vi "Cycle Diag Table Read.vi"(5 "Raw Data In":string) -> (4 "output cluster":T1)   [LabVIEW 2016, in "2015 VA Washer.lvlib"]
uses:
  Projects/2015 VA Washer.lvlib
  type defs/Cycle_Diag_Teststand.ctl
panel:
  out "appended array":string[](array[string])
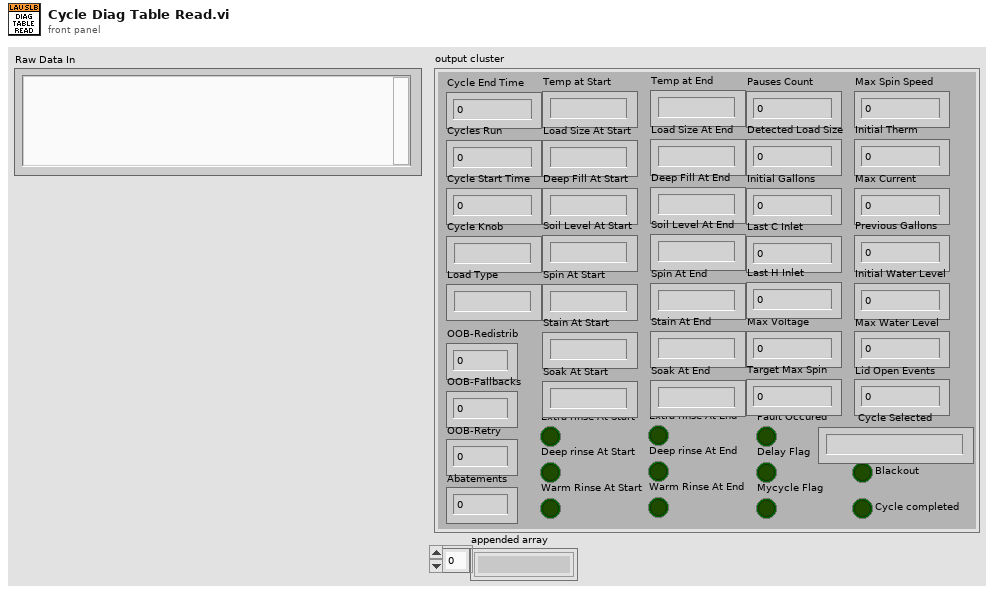
[diagram p1: front panel]
types:
  T1 = typedef "2015 VA Washer.lvlib/Cycle_Diag_Teststand.ctl" = cluster{"Cycle End Time":u32, "Cycles Run":u32, "Cycle Start Time":u32, "Cycle Knob":string, "Load Type":string, "OOB-Redistrib":u8, "OOB-Fallbacks":u8, "OOB-Retry":u8, "Temp at Start":string, "Load Size At Start":string, "Deep Fill At Start":string, "Soil Level At Start":string, "Spin At Start":string, "Extra rinse At Start":bool, "Deep rinse At Start":bool, "Stain At Start":string, "Soak At Start":string, "Warm Rinse At Start":bool, "Temp at End":string, "Load Size At End":string, "Deep Fill At End":string, "Soil Level At End":string, "Spin At End":string, "Extra rinse At End":bool, "Deep rinse At End":bool, "Stain At End":string, "Soak At End":string, "Warm Rinse At End":bool, "Pauses Count":u8, "Fault Occured":bool, "Delay Flag":bool, "Mycycle Flag":bool, "Blackout":bool, "Cycle completed":bool, "Detected Load Size":dbl, "Initial Gallons":dbl, "Last C Inlet ":dbl, "Max Voltage":dbl, "Target Max Spin":u16, "Max Spin Speed":u16, "Initial Therm":dbl, "Max Current":dbl, "Previous Gallons":dbl, "Initial Water Level":dbl, "Max Water Level":dbl, "Abatements ":u8, "Lid Open Events":u8, "Cycle Selected":string, "Last H Inlet ":dbl}
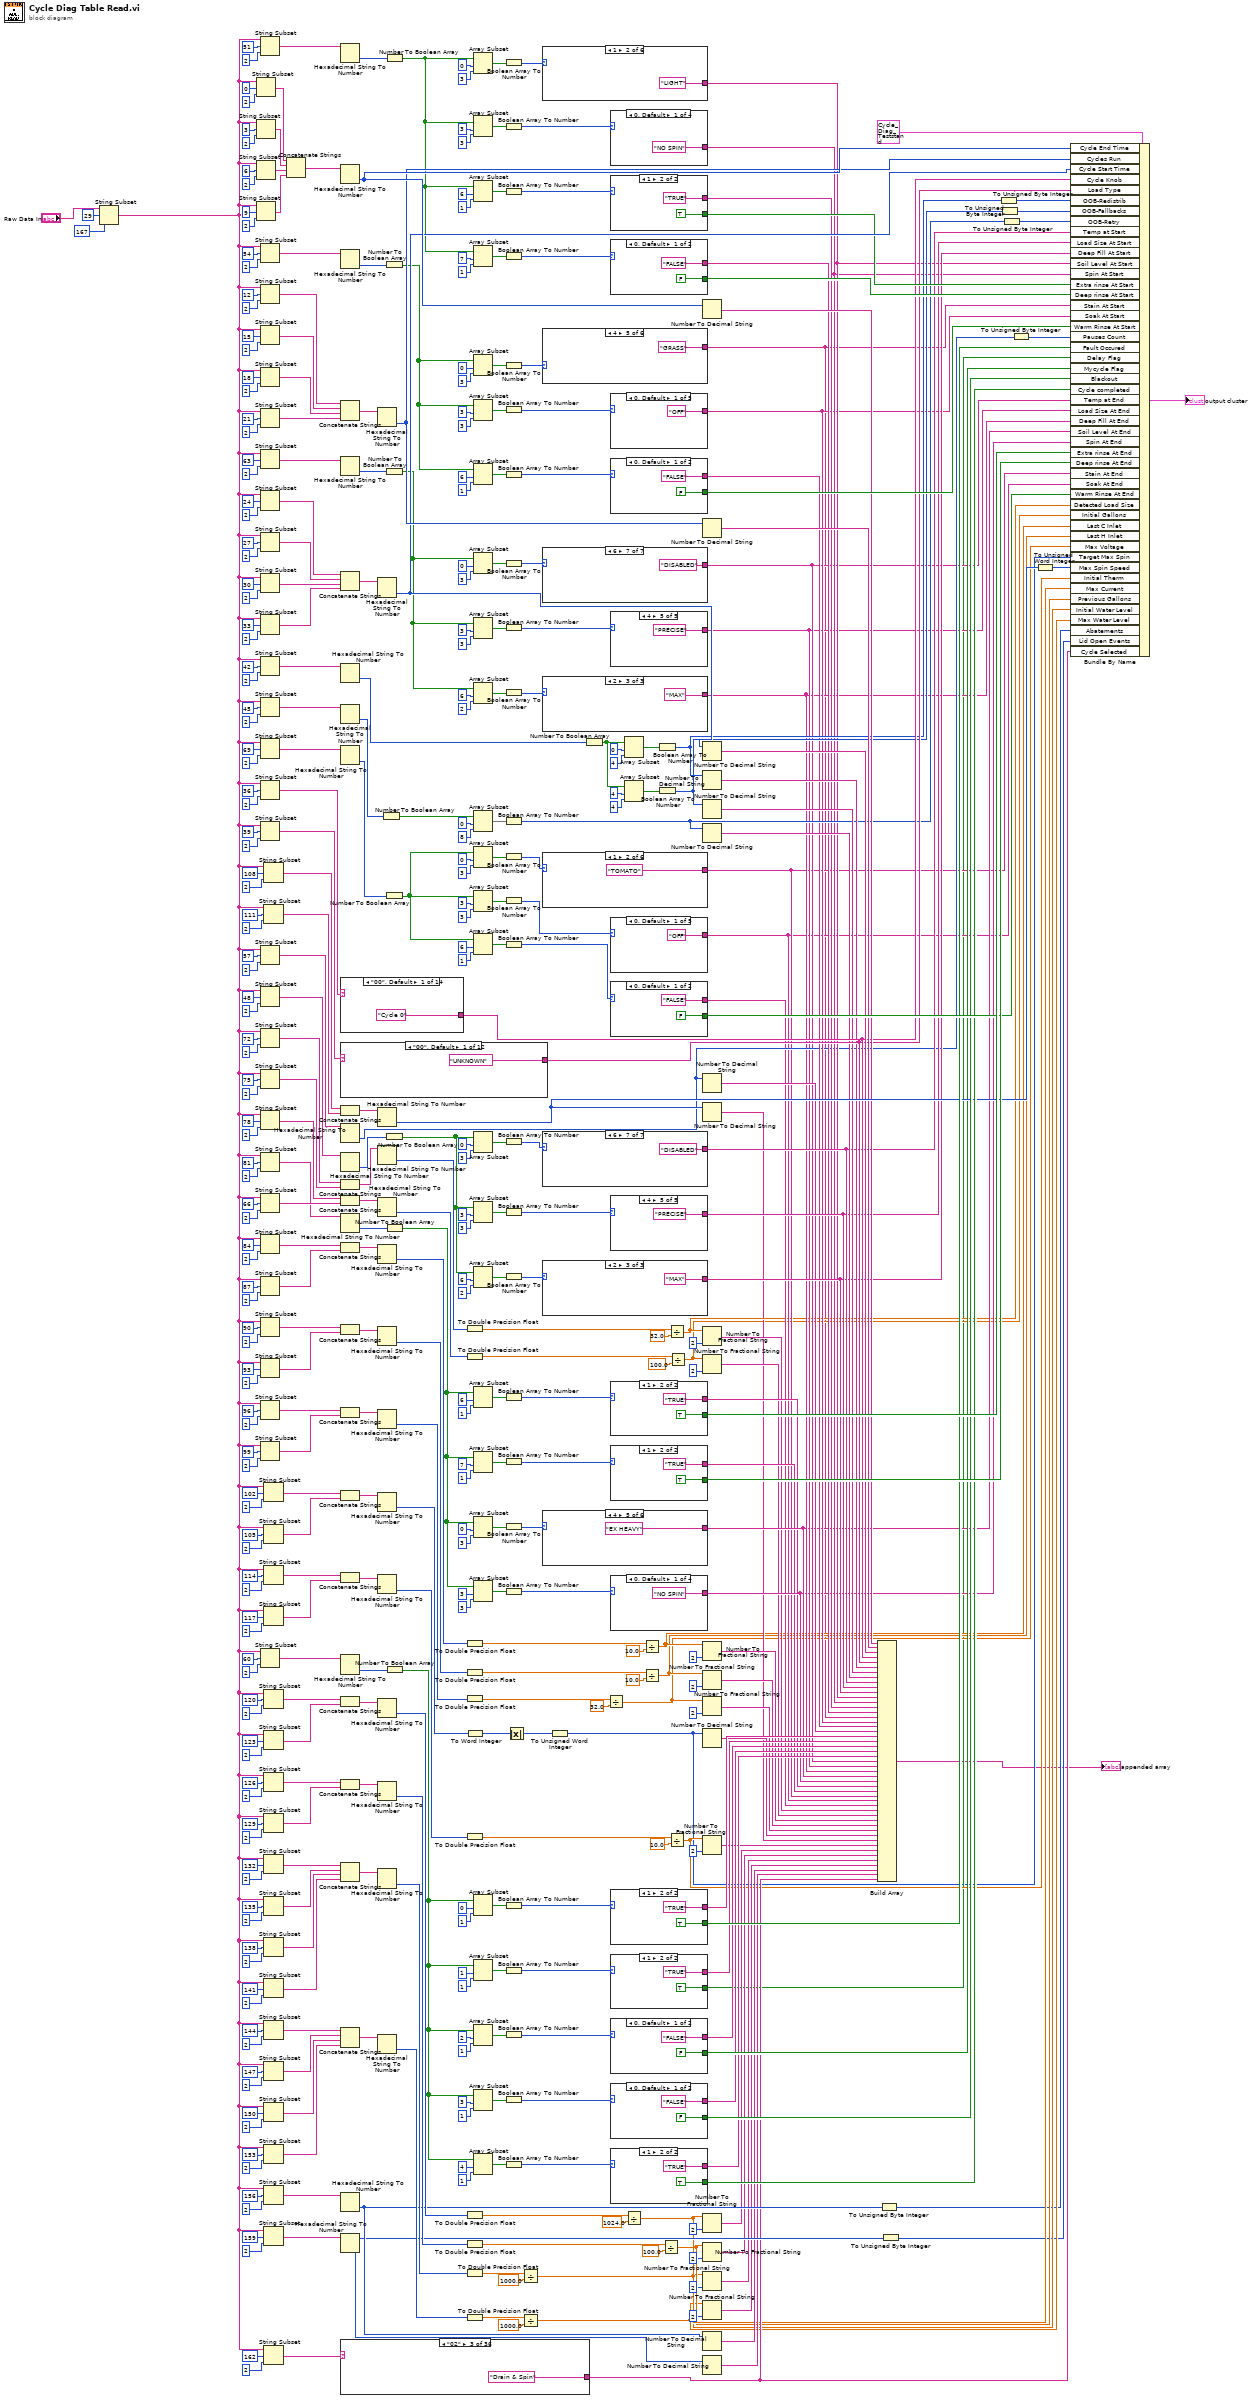
[diagram p0: block diagram]
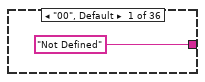
[diagram p2: hidden frame]
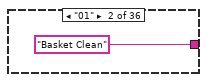
[diagram p3: hidden frame]
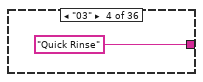
[diagram p4: hidden frame]
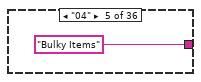
[diagram p5: hidden frame]
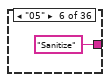
[diagram p6: hidden frame]
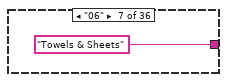
[diagram p7: hidden frame]
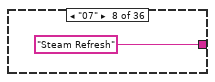
[diagram p8: hidden frame]
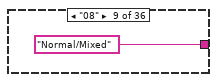
[diagram p9: hidden frame]
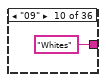
[diagram p10: hidden frame]
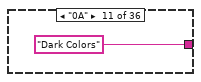
[diagram p11: hidden frame]
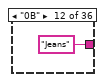
[diagram p12: hidden frame]
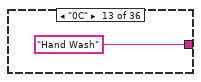
[diagram p13: hidden frame]
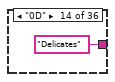
[diagram p14: hidden frame]
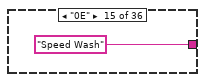
[diagram p15: hidden frame]
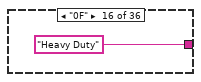
[diagram p16: hidden frame]
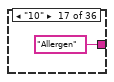
[diagram p17: hidden frame]
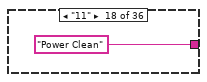
[diagram p18: hidden frame]
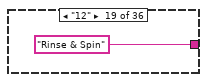
[diagram p19: hidden frame]
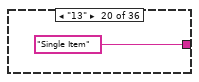
[diagram p20: hidden frame]
diagram:
  n1 = String Subset(string="Raw Data In", offset (0)=29, length (rest)=167 ("length (rest)")) -> (substring=w4:string)
  n2 = String Subset(string=w4, offset (0)=0, length (rest)=2 ("length (rest)")) -> (substring=w413:string)
  n3 = String Subset(string=w4, offset (0)=3, length (rest)=2 ("length (rest)")) -> (substring=w412:string)
  n4 = String Subset(string=w4, offset (0)=6, length (rest)=2 ("length (rest)")) -> (substring=w411:string)
  n5 = String Subset(string=w4, offset (0)=9, length (rest)=2 ("length (rest)")) -> (substring=w410:string)
  n6 = String Subset(string=w4, offset (0)=51, length (rest)=2 ("length (rest)")) -> (substring=w116:string)
  n7 = String Subset(string=w4, offset (0)=54, length (rest)=2 ("length (rest)")) -> (substring=w100:string)
  n8 = String Subset(string=w4, offset (0)=12, length (rest)=2 ("length (rest)")) -> (substring=w407:string)
  n9 = String Subset(string=w4, offset (0)=15, length (rest)=2 ("length (rest)")) -> (substring=w406:string)
  n10 = String Subset(string=w4, offset (0)=18, length (rest)=2 ("length (rest)")) -> (substring=w405:string)
  n11 = String Subset(string=w4, offset (0)=21, length (rest)=2 ("length (rest)")) -> (substring=w404:string)
  n12 = String Subset(string=w4, offset (0)=63, length (rest)=2 ("length (rest)")) -> (substring=w87:string)
  n13 = String Subset(string=w4, offset (0)=24, length (rest)=2 ("length (rest)")) -> (substring=w401:string)
  n14 = String Subset(string=w4, offset (0)=27, length (rest)=2 ("length (rest)")) -> (substring=w400:string)
  n15 = String Subset(string=w4, offset (0)=30, length (rest)=2 ("length (rest)")) -> (substring=w399:string)
  n16 = String Subset(string=w4, offset (0)=33, length (rest)=2 ("length (rest)")) -> (substring=w398:string)
  n17 = String Subset(string=w4, offset (0)=42, length (rest)=2 ("length (rest)")) -> (substring=w56:string)
  n18 = String Subset(string=w4, offset (0)=45, length (rest)=2 ("length (rest)")) -> (substring=w47:string)
  n19 = String Subset(string=w4, offset (0)=69, length (rest)=2 ("length (rest)")) -> (substring=w60:string)
  n20 = String Subset(string=w4, offset (0)=36, length (rest)=2 ("length (rest)")) -> (substring=w395:string)
  n21 = String Subset(string=w4, offset (0)=39, length (rest)=2 ("length (rest)")) -> (substring=w394:string)
  n22 = String Subset(string=w4, offset (0)=57, length (rest)=2 ("length (rest)")) -> (substring=w352:string)
  n23 = String Subset(string=w4, offset (0)=48, length (rest)=2 ("length (rest)")) -> (substring=w135:string)
  n24 = String Subset(string=w4, offset (0)=72, length (rest)=2 ("length (rest)")) -> (substring=w336:string)
  n25 = String Subset(string=w4, offset (0)=75 ("offset"), length (rest)=u32 2 ("default (0 U32)")) -> (substring=w333:string)
  n26 = String Subset(string=w4, offset (0)=78, length (rest)=2 ("length (rest)")) -> (substring=w328:string)
  n27 = String Subset(string=w4, offset (0)=81, length (rest)=2 ("length (rest)")) -> (substring=w327:string)
  n28 = String Subset(string=w4, offset (0)=66, length (rest)=2 ("length (rest)")) -> (substring=w73:string)
  n29 = String Subset(string=w4, offset (0)=84, length (rest)=2 ("length (rest)")) -> (substring=w317:string)
  n30 = String Subset(string=w4, offset (0)=87, length (rest)=2 ("length (rest)")) -> (substring=w316:string)
  n31 = String Subset(string=w4, offset (0)=90, length (rest)=2 ("length (rest)")) -> (substring=w311:string)
  n32 = String Subset(string=w4, offset (0)=93, length (rest)=2 ("length (rest)")) -> (substring=w310:string)
  n33 = String Subset(string=w4, offset (0)=96, length (rest)=2 ("length (rest)")) -> (substring=w301:string)
  n34 = String Subset(string=w4, offset (0)=99, length (rest)=2 ("length (rest)")) -> (substring=w300:string)
  n35 = String Subset(string=w4, offset (0)=60, length (rest)=2 ("length (rest)")) -> (substring=w351:string)
  n36 = String Subset(string=w4, offset (0)=108, length (rest)=2 ("length (rest)")) -> (substring=w288:string)
  n37 = String Subset(string=w4, offset (0)=111, length (rest)=2 ("length (rest)")) -> (substring=w287:string)
  n38 = String Subset(string=w4, offset (0)=102, length (rest)=2 ("length (rest)")) -> (substring=w291:string)
  n39 = String Subset(string=w4, offset (0)=105, length (rest)=2 ("length (rest)")) -> (substring=w290:string)
  n40 = String Subset(string=w4, offset (0)=114, length (rest)=2 ("length (rest)")) -> (substring=w276:string)
  n41 = String Subset(string=w4, offset (0)=117, length (rest)=2 ("length (rest)")) -> (substring=w275:string)
  n42 = String Subset(string=w4, offset (0)=120, length (rest)=2 ("length (rest)")) -> (substring=w266:string)
  n43 = String Subset(string=w4, offset (0)=123, length (rest)=2 ("length (rest)")) -> (substring=w265:string)
  n44 = String Subset(string=w4, offset (0)=126, length (rest)=2 ("length (rest)")) -> (substring=w256:string)
  n45 = String Subset(string=w4, offset (0)=129, length (rest)=2 ("length (rest)")) -> (substring=w255:string)
  n46 = String Subset(string=w4, offset (0)=132, length (rest)=2 ("length (rest)")) -> (substring=w246:string)
  n47 = String Subset(string=w4, offset (0)=135, length (rest)=2 ("length (rest)")) -> (substring=w245:string)
  n48 = String Subset(string=w4, offset (0)=138, length (rest)=2 ("length (rest)")) -> (substring=w215:string)
  n49 = String Subset(string=w4, offset (0)=141, length (rest)=2 ("length (rest)")) -> (substring=w214:string)
  n50 = String Subset(string=w4, offset (0)=144, length (rest)=2 ("length (rest)")) -> (substring=w240:string)
  n51 = String Subset(string=w4, offset (0)=147, length (rest)=2 ("length (rest)")) -> (substring=w239:string)
  n52 = String Subset(string=w4, offset (0)=150, length (rest)=2 ("length (rest)")) -> (substring=w209:string)
  n53 = String Subset(string=w4, offset (0)=153, length (rest)=2 ("length (rest)")) -> (substring=w208:string)
  n54 = String Subset(string=w4, offset (0)=156, length (rest)=2 ("length (rest)")) -> (substring=w220:string)
  n55 = String Subset(string=w4, offset (0)=159, length (rest)=2 ("length (rest)")) -> (substring=w219:string)
  n56 = String Subset(string=w4, offset (0)=162, length (rest)=2 ("length (rest)")) -> (substring=w216:string)
  n57 = Concatenate Strings(w413, w412, w411, w410) -> (w409:string)
  n58 = Hexadecimal String To Number(string=w116) -> (number=w123:u32)  [unwired: 2 in, 1 out]
  n59 = Hexadecimal String To Number(string=w409) -> (number=w408:u32)  [unwired: 2 in, 1 out]
  n60 = Hexadecimal String To Number(string=w100) -> (number=w108:u32)  [unwired: 2 in, 1 out]
  n61 = Concatenate Strings(w407, w406, w405, w404) -> (w403:string)
  n62 = Hexadecimal String To Number(string=w87) -> (number=w95:u32)  [unwired: 2 in, 1 out]
  n63 = Concatenate Strings(w401, w400, w399, w398) -> (w397:string)
  n64 = Hexadecimal String To Number(string=w56) -> (number=w55:u32)  [unwired: 2 in, 1 out]
  n65 = Hexadecimal String To Number(string=w47) -> (number=w46:u32)  [unwired: 2 in, 1 out]
  n66 = Hexadecimal String To Number(string=w60) -> (number=w68:u32)  [unwired: 2 in, 1 out]
  n67 = case shown="\"00\", Default" w395 {
    tunnel: ["Cycle 0" "Cycle 1" "Cycle 2" "Cycle 3" "Cycle 4" "Cycle 5" "Cycle 6" "Cycle 7" "Cycle 8" "Cycle 9" "Cycle 10" "Cycle 11" "Cycle 12" "Cycle 13"] -> w196
    frame "00", Default {
    }
    frame "01" {
    }
    frame "02" {
    }
    frame "03" {
    }
    frame "04" {
    }
    frame "05" {
    }
    frame "06" {
    }
    frame "07" {
    }
    frame "08" {
    }
    frame "09" {
    }
    frame "0A" {
    }
    frame "0B" {
    }
    frame "0C" {
    }
    frame "0D" {
    }
  }
  n68 = case shown="\"00\", Default" w394 {
    tunnel: ["UNKNOWN" "COTTON" "SYNTHETIC" "MIXED" "WET" "LOW FLOW" "SMALL" "MEDIUM" "LARGE" "SUPER" "SUPER PLUS" "MAX"] -> w195
    frame "00", Default {
    }
    frame "01" {
    }
    frame "02" {
    }
    frame "03" {
    }
    frame "04" {
    }
    frame "05" {
    }
    frame "06" {
    }
    frame "07" {
    }
    frame "08" {
    }
    frame "09" {
    }
    frame "0A" {
    }
    frame "0B" {
    }
  }
  n69 = Concatenate Strings(w288, w287) -> (w286:string)
  n70 = Hexadecimal String To Number(string=w352) -> (number=w179:u32)  [unwired: 2 in, 1 out]
  n71 = Hexadecimal String To Number(string=w135) -> (number=w134:u32)  [unwired: 2 in, 1 out]
  n72 = Concatenate Strings(w336, w333) -> (w332:string)
  n73 = Concatenate Strings(w328, w327) -> (w326:string)
  n74 = Hexadecimal String To Number(string=w73) -> (number=w83:u32)  [unwired: 2 in, 1 out]
  n75 = Concatenate Strings(w317, w316) -> (w315:string)
  n76 = Concatenate Strings(w311, w310) -> (w309:string)
  n77 = Concatenate Strings(w301, w300) -> (w299:string)
  n78 = Concatenate Strings(w291, w290) -> (w289:string)
  n79 = Concatenate Strings(w276, w275) -> (w274:string)
  n80 = Hexadecimal String To Number(string=w351) -> (number=w350:u32)  [unwired: 2 in, 1 out]
  n81 = Concatenate Strings(w266, w265) -> (w264:string)
  n82 = Concatenate Strings(w256, w255) -> (w254:string)
  n83 = Concatenate Strings(w246, w245, w215, w214) -> (w244:string)
  n84 = Concatenate Strings(w240, w239, w209, w208) -> (w238:string)
  n85 = Hexadecimal String To Number(string=w220) -> (number=w218:u32)  [unwired: 2 in, 1 out]
  n86 = Hexadecimal String To Number(string=w219) -> (number=w217:u32)  [unwired: 2 in, 1 out]
  n87 = case shown="\"02\"" w216 {
    tunnel: ["Not Defined" "Basket Clean" "Drain & Spin" "Quick Rinse" "Bulky Items" "Sanitize" "Towels & Sheets" "Steam Refresh" "Normal/Mixed" "Whites" "Dark Colors" "Jeans" "Hand Wash" "Delicates" "Speed Wash" "Heavy Duty" "Allergen" "Power Clean" "Rinse & Spin" "Single Item" "Colors" "Cold Wash" "Cottons" "Easy Care" "Active Wear" "Timed Dry" "Dewrinkle" "Air Fluff" "Steam Refresh" "Steam Dewrinkle" "Speed Dry" "Mixed" "Quick Dry" "Casuals" "Warm Up" "Energy Saver"] -> w146
    frame "00", Default {
    }
    frame "01" {
    }
    frame "02" {
    }
    frame "03" {
    }
    frame "04" {
    }
    frame "05" {
    }
    frame "06" {
    }
    frame "07" {
    }
    frame "08" {
    }
    frame "09" {
    }
    frame "0A" {
    }
    frame "0B" {
    }
    frame "0C" {
    }
    frame "0D" {
    }
    frame "0E" {
    }
    frame "0F" {
    }
    frame "10" {
    }
    frame "11" {
    }
    frame "12" {
    }
    frame "13" {
    }
    frame "14" {
    }
    frame "15" {
    }
    frame "80" {
    }
    frame "81" {
    }
    frame "82" {
    }
    frame "83" {
    }
    frame "84" {
    }
    frame "85" {
    }
    frame "86" {
    }
    frame "87" {
    }
    frame "88" {
    }
    frame "89" {
    }
    frame "8A" {
    }
    frame "8B" {
    }
    frame "8C" {
    }
    frame "8D" {
    }
  }
  n88 = Hexadecimal String To Number(string=w403) -> (number=w402:u32)  [unwired: 2 in, 1 out]
  n89 = Hexadecimal String To Number(string=w397) -> (number=w396:u32)  [unwired: 2 in, 1 out]
  n90 = Hexadecimal String To Number(string=w286) -> (number=w285:u32)  [unwired: 2 in, 1 out]
  n91 = Hexadecimal String To Number(string=w332) -> (number=w339:u32)  [unwired: 2 in, 1 out]
  n92 = Hexadecimal String To Number(string=w326) -> (number=w325:u32)  [unwired: 2 in, 1 out]
  n93 = Hexadecimal String To Number(string=w315) -> (number=w314:u32)  [unwired: 2 in, 1 out]
  n94 = Hexadecimal String To Number(string=w309) -> (number=w308:u32)  [unwired: 2 in, 1 out]
  n95 = Hexadecimal String To Number(string=w299) -> (number=w298:u32)  [unwired: 2 in, 1 out]
  n96 = Hexadecimal String To Number(string=w289) -> (number=w201:u32)  [unwired: 2 in, 1 out]
  n97 = Hexadecimal String To Number(string=w274) -> (number=w273:u32)  [unwired: 2 in, 1 out]
  n98 = Hexadecimal String To Number(string=w264) -> (number=w263:u32)  [unwired: 2 in, 1 out]
  n99 = Hexadecimal String To Number(string=w254) -> (number=w253:u32)  [unwired: 2 in, 1 out]
  n100 = Hexadecimal String To Number(string=w244) -> (number=w243:u32)  [unwired: 2 in, 1 out]
  n101 = Hexadecimal String To Number(string=w238) -> (number=w237:u32)  [unwired: 2 in, 1 out]
  n102 = Number To Boolean Array(number=w46) -> (Boolean array=w45:bool[])
  n103 = Number To Boolean Array(number=w108) -> (Boolean array=w107:bool[])
  n104 = Number To Boolean Array(number=w95) -> (Boolean array=w94:bool[])
  n105 = Number To Boolean Array(number=w68) -> (Boolean array=w67:bool[])
  n106 = Number To Boolean Array(number=w134) -> (Boolean array=w133:bool[])
  n107 = Number To Boolean Array(number=w123) -> (Boolean array=w115:bool[])
  n108 = Number To Boolean Array(number=w83) -> (Boolean array=w76:bool[])
  n109 = Number To Boolean Array(number=w350) -> (Boolean array=w31:bool[])
  n110 = To Double Precision Float(number=w339) -> (double precision float=w338:dbl)
  n111 = To Double Precision Float(number=w325) -> (double precision float=w324:dbl)
  n112 = To Double Precision Float(number=w314) -> (double precision float=w313:dbl)
  n113 = To Double Precision Float(number=w308) -> (double precision float=w307:dbl)
  n114 = To Double Precision Float(number=w298) -> (double precision float=w297:dbl)
  n115 = To Word Integer(number=w201) -> (16bit integer=w203:i16)
  n116 = To Double Precision Float(number=w273) -> (double precision float=w272:dbl)
  n117 = To Double Precision Float(number=w263) -> (double precision float=w262:dbl)
  n118 = To Double Precision Float(number=w253) -> (double precision float=w252:dbl)
  n119 = To Double Precision Float(number=w243) -> (double precision float=w242:dbl)
  n120 = To Double Precision Float(number=w237) -> (double precision float=w236:dbl)
  n121 = Array Subset(array=w115, index=0, length=3) -> (w112:bool[])
  n122 = Array Subset(array=w115, index=3, length=3) -> (w111:bool[])
  n123 = Array Subset(array=w115, index=6, length=1) -> (w110:bool[])
  n124 = Array Subset(array=w115, index=7, length=1) -> (w109:bool[])
  n125 = Array Subset(array=w107, index=0, length=3) -> (w98:bool[])
  n126 = Array Subset(array=w107, index=3, length=3) -> (w97:bool[])
  n127 = Array Subset(array=w107, index=6, length=1) -> (w96:bool[])
  n128 = Array Subset(array=w94, index=0, length=3) -> (w86:bool[])
  n129 = Array Subset(array=w94, index=3, length=3) -> (w85:bool[])
  n130 = Array Subset(array=w94, index=6, length=2) -> (w84:bool[])
  n131 = Array Subset(array=w45, index=0, length=8) -> (w42:bool[])
  n132 = Array Subset(array=w67, index=0, length=3) -> (w59:bool[])
  n133 = Array Subset(array=w67, index=3, length=3) -> (w58:bool[])
  n134 = Array Subset(array=w67, index=6, length=1) -> (w57:bool[])
  n135 = Array Subset(array=w133, index=0, length=3) -> (w126:bool[])
  n136 = Array Subset(array=w133, index=3, length=3) -> (w125:bool[])
  n137 = Array Subset(array=w133, index=6, length=2) -> (w124:bool[])
  n138 = Array Subset(array=w76, index=6, length=1) -> (w70:bool[])
  n139 = Array Subset(array=w76, index=7, length=1) -> (w69:bool[])
  n140 = Array Subset(array=w76, index=0, length=3) -> (w72:bool[])
  n141 = Array Subset(array=w76, index=3, length=3) -> (w71:bool[])
  n142 = Array Subset(array=w31, index=0, length=1) -> (w30:bool[])
  n143 = Array Subset(array=w31, index=1, length=1) -> (w28:bool[])
  n144 = Array Subset(array=w31, index=2, length=1) -> (w27:bool[])
  n145 = Array Subset(array=w31, index=3, length=1) -> (w26:bool[])
  n146 = Array Subset(array=w31, index=4, length=1) -> (w25:bool[])
  n147 = Boolean Array To Number(Boolean array=w112) -> (number=w385:u32)
  n148 = Boolean Array To Number(Boolean array=w111) -> (number=w384:u32)
  n149 = Boolean Array To Number(Boolean array=w110) -> (number=w383:u32)
  n150 = Boolean Array To Number(Boolean array=w109) -> (number=w382:u32)
  n151 = Boolean Array To Number(Boolean array=w98) -> (number=w379:u32)
  n152 = Boolean Array To Number(Boolean array=w97) -> (number=w378:u32)
  n153 = Boolean Array To Number(Boolean array=w96) -> (number=w377:u32)
  n154 = Boolean Array To Number(Boolean array=w86) -> (number=w369:u32)
  n155 = Boolean Array To Number(Boolean array=w85) -> (number=w368:u32)
  n156 = Boolean Array To Number(Boolean array=w84) -> (number=w367:u32)
  n157 = Boolean Array To Number(Boolean array=w42) -> (number=w189:u32)
  n158 = Boolean Array To Number(Boolean array=w59) -> (number=w362:u32)
  n159 = Boolean Array To Number(Boolean array=w58) -> (number=w361:u32)
  n160 = Boolean Array To Number(Boolean array=w57) -> (number=w360:u32)
  n161 = Boolean Array To Number(Boolean array=w126) -> (number=w200:u32)
  n162 = Boolean Array To Number(Boolean array=w125) -> (number=w387:u32)
  n163 = Boolean Array To Number(Boolean array=w124) -> (number=w386:u32)
  n164 = Boolean Array To Number(Boolean array=w70) -> (number=w364:u32)
  n165 = Boolean Array To Number(Boolean array=w69) -> (number=w363:u32)
  n166 = Boolean Array To Number(Boolean array=w72) -> (number=w366:u32)
  n167 = Boolean Array To Number(Boolean array=w71) -> (number=w365:u32)
  n168 = Boolean Array To Number(Boolean array=w30) -> (number=w349:u32)
  n169 = Boolean Array To Number(Boolean array=w28) -> (number=w348:u32)
  n170 = Boolean Array To Number(Boolean array=w27) -> (number=w347:u32)
  n171 = Boolean Array To Number(Boolean array=w26) -> (number=w346:u32)
  n172 = Boolean Array To Number(Boolean array=w25) -> (number=w345:u32)
  n173 = Absolute Value(x=w203) -> (abs(x)=w202:i16)
  n174 = Divide(x=w242, y=1000.0) -> (x/y=w139:dbl)
  n175 = Divide(x=w236, y=1000.0) -> (x/y=w138:dbl)
  n176 = case shown="1" w385 {
    tunnel: ["EXTRA LIGHT" "LIGHT" "NORMAL" "HEAVY" "EX HEAVY" "DISABLED"] -> w185
    frame 0, Default {
    }
    frame 1 {
    }
    frame 2 {
    }
    frame 3 {
    }
    frame 4 {
    }
    frame 5 {
    }
  }
  n177 = case shown="4" w379 {
    tunnel: ["OFF" "TOMATO" "WINE" "BLOOD" "GRASS" "DIRT"] -> w99
    frame 0, Default {
    }
    frame 1 {
    }
    frame 2 {
    }
    frame 3 {
    }
    frame 4 {
    }
    frame 5 {
    }
  }
  n178 = case shown="6" w369 {
    tunnel: ["TAP COLD" "COLD" "COOL" "COLORS" "WARM" "HOT" "DISABLED"] -> w171
    frame 0, Default {
    }
    frame 1 {
    }
    frame 2 {
    }
    frame 3 {
    }
    frame 4 {
    }
    frame 5 {
    }
    frame 6 {
    }
  }
  n179 = case shown="2" w367 {
    tunnel: ["OFF" "INCREMENTAL" "MAX"] -> w169
    frame 0, Default {
    }
    frame 1 {
    }
    frame 2 {
    }
  }
  n180 = case shown="1" w362 {
    tunnel: ["OFF" "TOMATO" "WINE" "BLOOD" "GRASS" "DIRT"] -> w164
    frame 0, Default {
    }
    frame 1 {
    }
    frame 2 {
    }
    frame 3 {
    }
    frame 4 {
    }
    frame 5 {
    }
  }
  n181 = case shown="6" w200 {
    tunnel: ["TAP COLD" "COLD" "COOL" "COLORS" "WARM" "HOT" "DISABLED"] -> w188
    frame 0, Default {
    }
    frame 1 {
    }
    frame 2 {
    }
    frame 3 {
    }
    frame 4 {
    }
    frame 5 {
    }
    frame 6 {
    }
  }
  n182 = case shown="2" w386 {
    tunnel: ["OFF" "INCREMENTAL" "MAX"] -> w186
    frame 0, Default {
    }
    frame 1 {
    }
    frame 2 {
    }
  }
  n183 = case shown="4" w366 {
    tunnel: ["EXTRA LIGHT" "LIGHT" "NORMAL" "HEAVY" "EX HEAVY" "DISABLED"] -> w168
    frame 0, Default {
    }
    frame 1 {
    }
    frame 2 {
    }
    frame 3 {
    }
    frame 4 {
    }
    frame 5 {
    }
  }
  n184 = To Unsigned Word Integer(number=w202) -> (unsigned 16bit integer=w14:u16)
  n185 = Number To Boolean Array(number=w55) -> (Boolean array=w50:bool[])
  n186 = Divide(x=w297, y=32.0) -> (x/y=w143:dbl)
  n187 = case shown="0, Default" w384 {
    tunnel: ["NO SPIN" "NORMAL" "MORE" "MAX"] -> w184
    frame 0, Default {
    }
    frame 1 {
    }
    frame 2 {
    }
    frame 3 {
    }
  }
  n188 = case shown="1" w383 {
    tunnel: [FALSE TRUE] -> w381
    tunnel: ["FALSE" "TRUE"] -> w183
    frame 0, Default {
    }
    frame 1 {
    }
  }
  n189 = case shown="0, Default" w382 {
    tunnel: [FALSE TRUE] -> w380
    tunnel: ["FALSE" "TRUE"] -> w182
    frame 0, Default {
    }
    frame 1 {
    }
  }
  n190 = case shown="0, Default" w378 {
    tunnel: ["OFF" "15 MIN" "30 MIN" "60 MIN" "2 HOURS"] -> w181
    frame 0, Default {
    }
    frame 1 {
    }
    frame 2 {
    }
    frame 3 {
    }
    frame 4 {
    }
  }
  n191 = case shown="0, Default" w377 {
    tunnel: [FALSE TRUE] -> w376
    tunnel: ["FALSE" "TRUE"] -> w180
    frame 0, Default {
    }
    frame 1 {
    }
  }
  n192 = case shown="4" w368 {
    tunnel: ["SMALL" "MEDIUM" "LARGE" "SUPER" "PRECISE"] -> w170
    frame 0, Default {
    }
    frame 1 {
    }
    frame 2 {
    }
    frame 3 {
    }
    frame 4 {
    }
  }
  n193 = case shown="0, Default" w361 {
    tunnel: ["OFF" "15 MIN" "30 MIN" "60 MIN" "2 HOURS"] -> w163
    frame 0, Default {
    }
    frame 1 {
    }
    frame 2 {
    }
    frame 3 {
    }
    frame 4 {
    }
  }
  n194 = case shown="0, Default" w360 {
    tunnel: [FALSE TRUE] -> w357
    tunnel: ["FALSE" "TRUE"] -> w162
    frame 0, Default {
    }
    frame 1 {
    }
  }
  n195 = case shown="4" w387 {
    tunnel: ["SMALL" "MEDIUM" "LARGE" "SUPER" "PRECISE"] -> w187
    frame 0, Default {
    }
    frame 1 {
    }
    frame 2 {
    }
    frame 3 {
    }
    frame 4 {
    }
  }
  n196 = case shown="1" w364 {
    tunnel: [FALSE TRUE] -> w359
    tunnel: ["FALSE" "TRUE"] -> w166
    frame 0, Default {
    }
    frame 1 {
    }
  }
  n197 = case shown="1" w363 {
    tunnel: [FALSE TRUE] -> w358
    tunnel: ["FALSE" "TRUE"] -> w165
    frame 0, Default {
    }
    frame 1 {
    }
  }
  n198 = case shown="0, Default" w365 {
    tunnel: ["NO SPIN" "NORMAL" "MORE" "MAX"] -> w167
    frame 0, Default {
    }
    frame 1 {
    }
    frame 2 {
    }
    frame 3 {
    }
  }
  n199 = case shown="1" w349 {
    tunnel: [FALSE TRUE] -> w344
    tunnel: ["FALSE" "TRUE"] -> w176
    frame 0, Default {
    }
    frame 1 {
    }
  }
  n200 = case shown="1" w348 {
    tunnel: [FALSE TRUE] -> w29
    tunnel: ["FALSE" "TRUE"] -> w175
    frame 0, Default {
    }
    frame 1 {
    }
  }
  n201 = case shown="0, Default" w347 {
    tunnel: [FALSE TRUE] -> w177
    tunnel: ["FALSE" "TRUE"] -> w174
    frame 0, Default {
    }
    frame 1 {
    }
  }
  n202 = case shown="0, Default" w346 {
    tunnel: [FALSE TRUE] -> w343
    tunnel: ["FALSE" "TRUE"] -> w173
    frame 0, Default {
    }
    frame 1 {
    }
  }
  n203 = case shown="1" w345 {
    tunnel: [FALSE TRUE] -> w342
    tunnel: ["FALSE" "TRUE"] -> w172
    frame 0, Default {
    }
    frame 1 {
    }
  }
  n204 = Array Subset(array=w50, index=0, length=4) -> (w49:bool[])
  n205 = Array Subset(array=w50, index=4, length=4) -> (w48:bool[])
  n206 = Divide(x=w262, y=1024.0) -> (x/y=w141:dbl)
  n207 = Divide(x=w313, y=10.0) -> (x/y=w145:dbl)
  n208 = Divide(x=w307, y=10.0) -> (x/y=w144:dbl)
  n209 = Boolean Array To Number(Boolean array=w49) -> (number=w194:u32)
  n210 = Boolean Array To Number(Boolean array=w48) -> (number=w192:u32)
  n211 = Divide(x=w252, y=100.0) -> (x/y=w140:dbl)
  n212 = Divide(x=w338, y=32.0) -> (x/y=w161:dbl)
  n213 = Divide(x=w272, y=10.0) -> (x/y=w142:dbl)
  n214 = Divide(x=w324, y=100.0) -> (x/y=w137:dbl)
  n215 = Number To Decimal String(number=w408) -> (decimal integer string=w199:string)  [unwired: 1 in]
  n216 = Number To Decimal String(number=w402) -> (decimal integer string=w198:string)  [unwired: 1 in]
  n217 = Number To Decimal String(number=w396) -> (decimal integer string=w197:string)  [unwired: 1 in]
  n218 = Number To Decimal String(number=w194) -> (decimal integer string=w193:string)  [unwired: 1 in]
  n219 = Number To Decimal String(number=w192) -> (decimal integer string=w191:string)  [unwired: 1 in]
  n220 = Number To Decimal String(number=w189) -> (decimal integer string=w190:string)  [unwired: 1 in]
  n221 = Number To Decimal String(number=w179) -> (decimal integer string=w178:string)  [unwired: 1 in]
  n222 = Number To Decimal String(number=w285) -> (decimal integer string=w154:string)  [unwired: 1 in]
  n223 = Number To Fractional String(number=w161, precision (6)=i16 2) -> (F-format string=w160:string)  [unwired: 2 in]
  n224 = Number To Fractional String(number=w137, precision (6)=i16 2) -> (F-format string=w159:string)  [unwired: 2 in]
  n225 = Number To Fractional String(number=w145, precision (6)=i16 2) -> (F-format string=w158:string)  [unwired: 2 in]
  n226 = Number To Fractional String(number=w144, precision (6)=i16 2) -> (F-format string=w157:string)  [unwired: 2 in]
  n227 = Number To Fractional String(number=w143, precision (6)=i16 2) -> (F-format string=w156:string)  [unwired: 2 in]
  n228 = Number To Decimal String(number=w14) -> (decimal integer string=w155:string)  [unwired: 1 in]
  n229 = Number To Fractional String(number=w142, precision (6)=i16 2) -> (F-format string=w153:string)  [unwired: 2 in]
  n230 = Number To Fractional String(number=w141, precision (6)=i16 2) -> (F-format string=w152:string)  [unwired: 2 in]
  n231 = Number To Fractional String(number=w140, precision (6)=i16 2) -> (F-format string=w151:string)  [unwired: 2 in]
  n232 = Number To Fractional String(number=w139, precision (6)=i16 2) -> (F-format string=w150:string)  [unwired: 2 in]
  n233 = Number To Fractional String(number=w138, precision (6)=i16 2) -> (F-format string=w149:string)  [unwired: 2 in]
  n234 = Number To Decimal String(number=w218) -> (decimal integer string=w148:string)  [unwired: 1 in]
  n235 = Number To Decimal String(number=w217) -> (decimal integer string=w147:string)  [unwired: 1 in]
  n236 = Build Array(w199, w198, w197, w196, w195, w193, w191, w190, w188, w187, w186, w185, w184, w183, w182, w99, w181, w180, w178, w176, w175, w174, w173, w172, w171, w170, w169, w168, w167, w166, w165, w164, w163, w162, w160, w159, w158, w157, w156, w155, w154, w153, w152, w151, w150, w149, w148, w147, w146) -> (→"appended array":string[])
  n237 = To Unsigned Byte Integer(number=w218) -> (unsigned 8bit integer=w13:u8)
  n238 = To Unsigned Byte Integer(number=w217) -> (unsigned 8bit integer=w12:u8)
  n239 = To Unsigned Byte Integer(number=w194) -> (unsigned 8bit integer=w24:u8)
  n240 = To Unsigned Byte Integer(number=w192) -> (unsigned 8bit integer=w23:u8)
  n241 = To Unsigned Byte Integer(number=w189) -> (unsigned 8bit integer=w22:u8)
  n242 = To Unsigned Byte Integer(number=w179) -> (unsigned 8bit integer=w21:u8)
  n243 = To Unsigned Word Integer(number=w285) -> (unsigned 16bit integer=w15:u16)
  n244 = Bundle By Name(cluster=T1 {"Cycle End Time"=0, "Cycles Run"=0, "Cycle Start Time"=0, "Cycle Knob"="", "Load Type"="", "OOB-Redistrib"=0, "OOB-Fallbacks"=0, "OOB-Retry"=0, "Temp at Start"="", "Load Size At Start"="", "Deep Fill At Start"="", "Soil Level At Start"="", "Spin At Start"="", "Extra rinse At Start"=FALSE, "Deep rinse At Start"=FALSE, "Stain At Start"="", "Soak At Start"="", "Warm Rinse At Start"=FALSE, "Temp at End"="", "Load Size At End"="", "Deep Fill At End"="", "Soil Level At End"="", "Spin At End"="", "Extra rinse At End"=FALSE, "Deep rinse At End"=FALSE, "Stain At End"="", "Soak At End"="", "Warm Rinse At End"=FALSE, "Pauses Count"=0, "Fault Occured"=FALSE, "Delay Flag"=FALSE, "Mycycle Flag"=FALSE, "Blackout"=FALSE, "Cycle completed"=FALSE, "Detected Load Size"=0.0, "Initial Gallons"=0.0, "Last C Inlet "=0.0, "Max Voltage"=0.0, "Target Max Spin"=0, "Max Spin Speed"=0, "Initial Therm"=0.0, "Max Current"=0.0, "Previous Gallons"=0.0, "Initial Water Level"=0.0, "Max Water Level"=0.0, "Abatements "=0, "Lid Open Events"=0, "Cycle Selected"="", "Last H Inlet "=0.0} ("Cycle History Diagnostics"), "Cycle End Time"=w408, "Cycles Run"=w402, "Cycle Start Time"=w396, "Cycle Knob"=w196, "Load Type"=w195, "OOB-Redistrib"=w24, "OOB-Fallbacks"=w23, "OOB-Retry"=w22, "Temp at Start"=w188, "Load Size At Start"=w187, "Deep Fill At Start"=w186, "Soil Level At Start"=w185, "Spin At Start"=w184, "Extra rinse At Start"=w381, "Deep rinse At Start"=w380, "Stain At Start"=w99, "Soak At Start"=w181, "Warm Rinse At Start"=w376, "Pauses Count"=w21, "Fault Occured"=w344, "Delay Flag"=w29, "Mycycle Flag"=w177, "Blackout"=w343, "Cycle completed"=w342, "Temp at End"=w171, "Load Size At End"=w170, "Deep Fill At End"=w169, "Soil Level At End"=w168, "Spin At End"=w167, "Extra rinse At End"=w359, "Deep rinse At End"=w358, "Stain At End"=w164, "Soak At End"=w163, "Warm Rinse At End"=w357, "Detected Load Size"=w161, "Initial Gallons"=w137, "Last C Inlet"=w145, "Last H Inlet"=w144, "Max Voltage"=w143, "Target Max Spin"=w14, "Max Spin Speed"=w15, "Initial Therm"=w142, "Max Current"=w141, "Previous Gallons"=w140, "Initial Water Level"=w139, "Max Water Level"=w138, "Abatements"=w13, "Lid Open Events"=w12, "Cycle Selected"=w146) -> (→"output cluster":T1)
